vi "Error Cluster Generator.vi"(4 "error in":errorcluster, 5 "Error (T)":bool=TRUE, 6 "code":i32, 7 "Additional message":string) -> (1 "error out":errorcluster, 2 "Error Out":bool)   [LabVIEW 2018]
doc: "Error Cluster Generator.vi\n\nThis VI returns an error cluster for its calling VI with its calling VI's chain as a single string. No error cluster is generated if the Code input is zero or the Error In cluster contains an error. This version only creates an error if the Error? input is True. It does not create warnings. This allows for this VI to be placed in-line with error chains more easily.\n\nOCC Streaming Data System Version 1.0\nAugust, 2007 Original Code Consulting David Thomson\n www.originalcode.com"
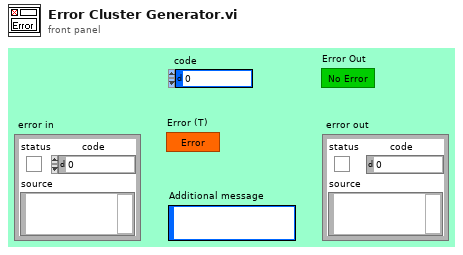
[diagram p1: front panel]
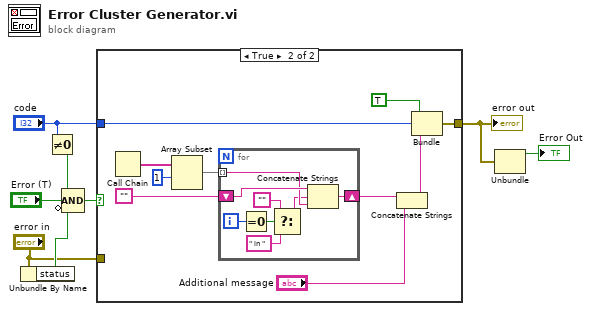
[diagram p0: block diagram]
diagram:
  n1 = Unbundle By Name("error in") -> ("status"=w5:bool)
  n2 = Not Equal To 0?(x="code") -> (x != 0?=w4:bool)
  n3 = Compound Arithmetic op=AND(w4, "Error (T)", invert w5) -> (w3:bool)
  n4 = case shown="True" w3 {
    tunnel: [w9 w19] -> w7
    tunnel: "code" -> [_ w18]
    tunnel: "error in" -> [w9 _]
    frame False {
    }
    frame True {
      n5 = Call Chain() -> (call chain=w16:string[])
      n6 = Array Subset(array=w16, index=1) -> (w14:string[])  [unwired: 1 in]
      n7 = for {
        tunnel: w14 -> [w24] mode=indexing
        shift-right: [w26] -> w13
        shift-left: "" -> [w27]
        i -> [w25]
        n8 = Equal To 0?(x=w25) -> (x = 0?=w22:bool)
        n9 = Select(t="", s=w22, f=" in ") -> (s? t:f=w23:string)
        n10 = Concatenate Strings(w27, w23, w24) -> (w26:string)
      }
      n11 = Concatenate Strings(w13, "Additional message") -> (w11:string)
      n12 = Bundle(TRUE, "code"=w18, w11) -> (w19:cluster{bool, "code":i32, string})  [unwired: 1 out]
    }
  }
  "error out" <- w7
  n13 = Unbundle(w7) -> ("status"=→"Error Out":bool)  [unwired: 2 out]
